vi "dsdll_capture_wave_auto_float32.vi"(8 "error in":errorcluster, 9 "transpose (false)":bool, 10 "samples count in":u32, 11 "dsdll instance in":T1={"dsdll path"=path "E:/LVprog/DirectSoundDLL/dsdll.dll", "dsdll handle"=[], "output devices"=[], "capture devices"=[]}) -> (0 "error out":errorcluster, 1 "float32 waves":sgl[][](array[numeric]), 2 "samples count out":u32, 3 "dsdll instance out":T1, 4 "channels count":i32, 5 "time stamp [s]":dbl)   [LabVIEW 2020, in "dsdll.lvlib"]
doc: "Call this to capture waveform of specified length.\nThis VI si synchronous so it won't return untill entire waveform is recorded.\n\nOutput is always float32 independent to actual capture format. Samples are normalized to <-1;1> range. Array organization:\n'transpose' = false: row = channels, columns = samples\n'transpose' = true: column = channels, rows = samples"
uses:
  dsdll.lvlib
  dsdll_instance.ctl
  dsdll_device_record.ctl
panel:
  out "variant sample data":variant
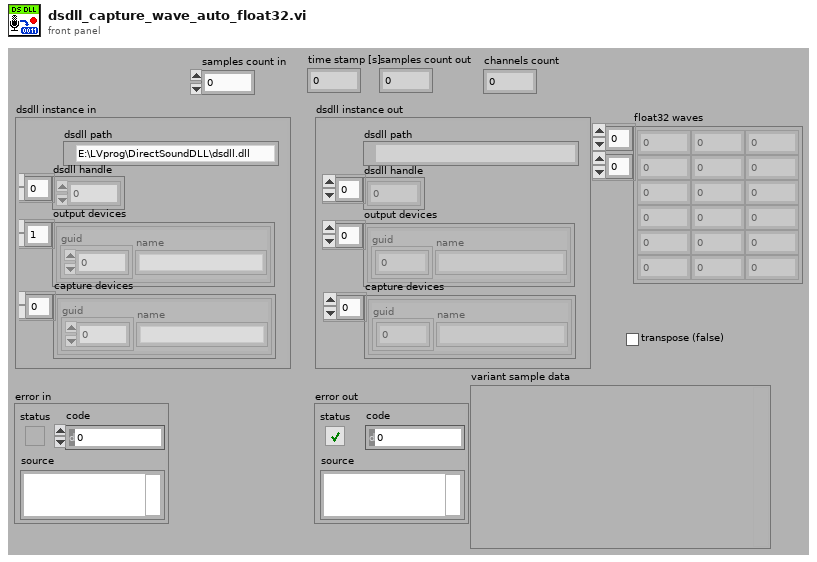
[diagram p1: front panel]
types:
  T1 = typedef "dsdll.lvlib/dsdll_instance.ctl" = cluster{"dsdll path":path, "dsdll handle":u8[], "output devices":T2[], "capture devices":T2[]}
  T2 = typedef "dsdll.lvlib/dsdll_device_record.ctl" = cluster{"guid":u8[], "name":string}
  T3 = typedef "dsdll.lvlib/dsdll_sample_format.ctl" = enum16{"IEEE float 32", "PCM 16 bit"}
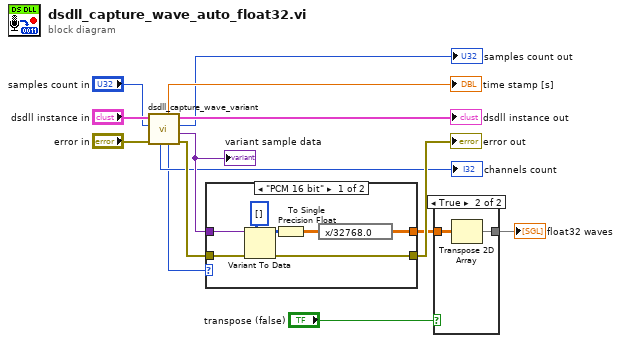
[diagram p0: block diagram]
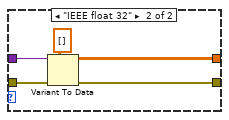
[diagram p2: hidden frame]
diagram:
  n1 = call "dsdll_capture_wave_variant.vi"("error in"="error in", "samples count in"="samples count in", "dsdll instance in"="dsdll instance in") -> ("error out"=w6:errorcluster, "variant sample data"=w4:variant, "samples count out"=→"samples count out":u32, "dsdll instance out"=→"dsdll instance out":T1, "format"=w1:T3, "time stamp [s]"=→"time stamp [s]":dbl, "channels count"=→"channels count":u16)  [unwired: 2 in]
  "variant sample data" <- w4
  n2 = case shown="\"PCM 16 bit\"" w1 {
    tunnel: w6 -> [w21 w26]
    tunnel: [w20 w25] -> w5
    tunnel: w4 -> [w16 w24]
    tunnel: [w15 w23] -> w3
    frame "PCM 16 bit" {
      n3 = Variant To Data(error in=w21, type=i16[][] [], Variant=w16) -> (data=w19:i16[][], error out=w20:errorcluster)
      n4 = To Single Precision Float(number=w19) -> (single precision float=w17:sgl[][])
      n5 = expression code="x/32768.0"(w17) -> (w15:sgl[][])
    }
    frame "IEEE float 32" {
      n6 = Variant To Data(error in=w26, type=sgl[][] [], Variant=w24) -> (data=w23:sgl[][], error out=w25:errorcluster)
    }
  }
  "error out" <- w5
  n7 = case shown="True" "transpose (false)" {
    tunnel: w3 -> [w27 w29]
    tunnel: [w27 w28] -> w9
    frame False {
    }
    frame True {
      n8 = Transpose 2D Array(2D array=w29) -> (transposed array=w28:sgl[][])
    }
  }
  "float32 waves" <- w9
